vi "NXT-M Hold Position.vi"() -> ()   [LabVIEW 2010]
uses:
  <vilib>/NXT/Subs/MotorOutput.ctl
  <vilib>/NXT/Subs/LVHSConnector.ctl
  <vilib>/NXT/Dual Mode Library/prims/inRangeAndCoerce/inRangeAndCoerce_int.vi
  <vilib>/NXT/Dual Mode Library/Motors/MotorOn.vi
panel:
  in  "NXT 2":T1
  out "NXT":T1
  in  "Output Port (All Ports)":T2=3 items=["Port A"=0, "Port B"=1, "Port C"=2, "Ports A & B"=4, "Ports A & C"=5, "Ports B & C"=6, "All Ports"=3]
  in  "Port (Port A)":u8(ring) items=["Port A", "Port B", "Port C"]
  in  "x":i32
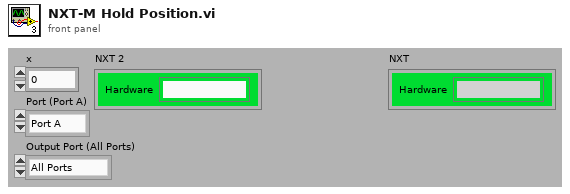
[diagram p1: front panel]
types:
  T1 = typedef "LVHSConnector.ctl" = cluster{"Hardware":string, "Flattened String":string}
  T2 = typedef "MotorOutput.ctl" = u8
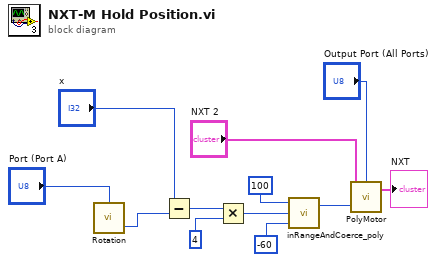
[diagram p0: block diagram]
diagram:
  n1 = call <vilib>:"Rotation.vi"("Port (Port A)"="Port (Port A)") -> ("Angle of Rotation"=w6:i32)  [unwired: 2 in, 1 out]
  n2 = Subtract(x="x", y=w6) -> (x-y=w7:i32)
  n3 = Multiply(x=w7, y=4) -> (x*y=w8:i32)
  n4 = call-poly <vilib>:"inRangeAndCoerce_poly.vi"("lower limit"=-60, "x"=w8, "upper limit"=100) -> ("coerced(x)"=w11:i32)  [unwired: 1 out]
  n5 = call-poly <vilib>:"PolyMotor.vi"("Power (75)"=w11, "NXT"="NXT 2", "Output Port (All Ports)"="Output Port (All Ports)") -> ("NXT"=→"NXT":T1)  [unwired: 1 in]
